vi "U8-U16.vi"(1 "数组":u8[](array[numeric]), 3 "error in (no error)":errorcluster caption="错误输入（无错误）") -> (8 "16位整型":u16, 10 "error out":errorcluster caption="错误输出")   [LabVIEW 2014]
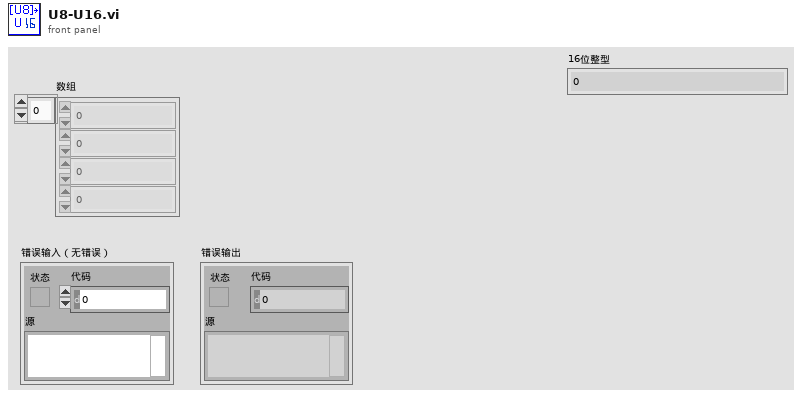
[diagram p1: front panel]
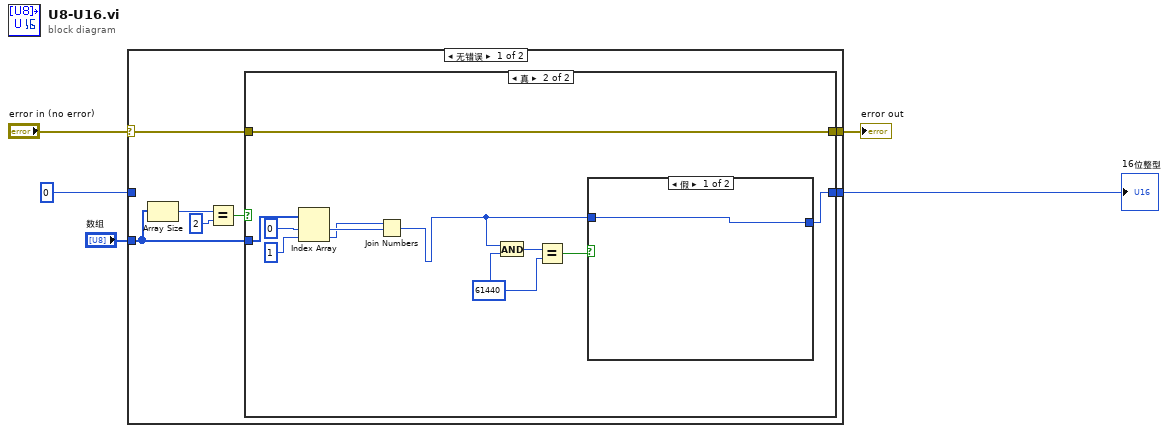
[diagram p0: block diagram]
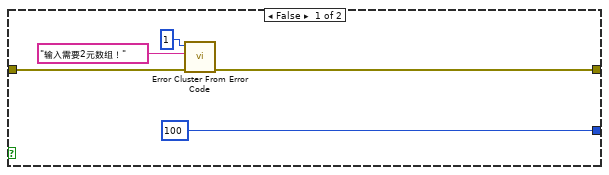
[diagram p2: hidden frame]
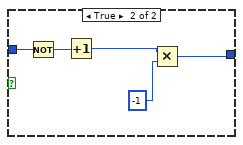
[diagram p3: hidden frame]
diagram:
  n1 = case shown="无错误" "error in (no error)" {
    selector: "error in (no error)" -> [w12 w36]
    tunnel: [w11 w36] -> w4
    tunnel: "数组" -> [w7 _]
    tunnel: 0 -> [_ w35]
    tunnel: [w6 w35] -> w1
    frame No Error {
      n2 = Array Size(array=w7) -> (size(s)=w10:i32)
      n3 = Equal?(x=w10, y=2) -> (x = y?=w8:bool)
      n4 = case shown="真" w8 {
        tunnel: w12 -> [w15 w25]
        tunnel: [w14 w25] -> w11
        tunnel: w7 -> [_ w26]
        tunnel: [100 w21] -> w6
        frame False {
          n5 = call <vilib>:"Error Cluster From Error Code.vi"("error in (no error)"=w15, "error message (\"\")"="输入需要2元数组！" ("error message (\"\")"), "error code (0)"=1) -> ("error out"=w14:errorcluster)  [unwired: 6 in]
        }
        frame True {
          w23 = 61440 ("y")
          n6 = Index Array(array=w26, index #1=0 ("索引"), index #2=1 ("索引")) -> (element #1=w19:u8, element #2=w18:u8)
          n7 = Join Numbers(hi=w18, lo=w19) -> ((hi.lo)=w20:u16)
          n8 = And(x=w20, y=w23) -> (x .and. y?=w24:i32)
          n9 = Equal?(x=w24, y=w23) -> (x = y?=w22:bool)
          n10 = case shown="假" w22 {
            tunnel: w20 -> [w29 w33]
            tunnel: [w29 w31] -> w21
            frame False {
            }
            frame True {
              n11 = Not(x=w33) -> (.not. x?=w34:u16)
              n12 = Increment(x=w34) -> (x+1=w30:u16)
              n13 = Multiply(x=w30, y=-1) -> (x*y=w31:i32)
            }
          }
        }
      }
    }
    frame Error {
    }
  }
  "error out" <- w4
  "16位整型" <- w1
